vi "Read NI.LV.Dialog Instance.vi"(11 "Project Stuff in":refnum<class "Project Stuff.lvclass">) -> (2 "NI.LV.Dialog Instance":refnum<vi>)   [LabVIEW 2020, in "_Shared.lvlib" / "Project Stuff.lvclass"]
uses:
  Project Stuff.lvclass
  Project Stuff.lvclass/Project Stuff.ctl
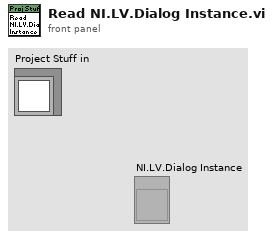
[diagram p1: front panel]
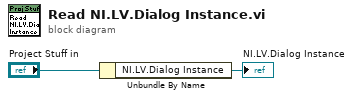
[diagram p0: block diagram]
diagram:
  n1 = Unbundle By Name("Project Stuff in") -> ("NI.LV.Dialog Instance"=→"NI.LV.Dialog Instance":refnum<vi>)
